vi "GPS init.vi"(11 "VISA resource name in":refnum<visa-resource-name>) -> (3 "VISA resource name out":refnum<visa-resource-name>)   [LabVIEW 2014]
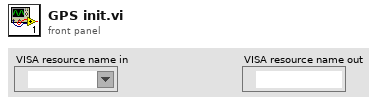
[diagram p1: front panel]
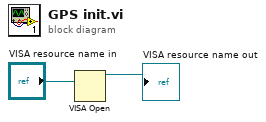
[diagram p0: block diagram]
diagram:
  n1 = VISA Open(VISA resource name="VISA resource name in") -> (VISA resource name=→"VISA resource name out":refnum<visa-resource-name>)  [unwired: 4 in, 1 out]
